vi "Run Explain Error.vi"(8 "error in (no error)":errorcluster, 11 "Data":errorcluster) -> (0 "error out":errorcluster)   [LabVIEW 2011, in "Simple Error Out.xctl"]
uses:
  Simple Error Out.xctl
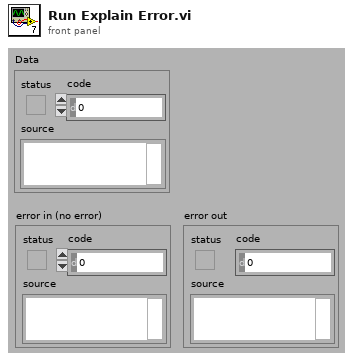
[diagram p1: front panel]
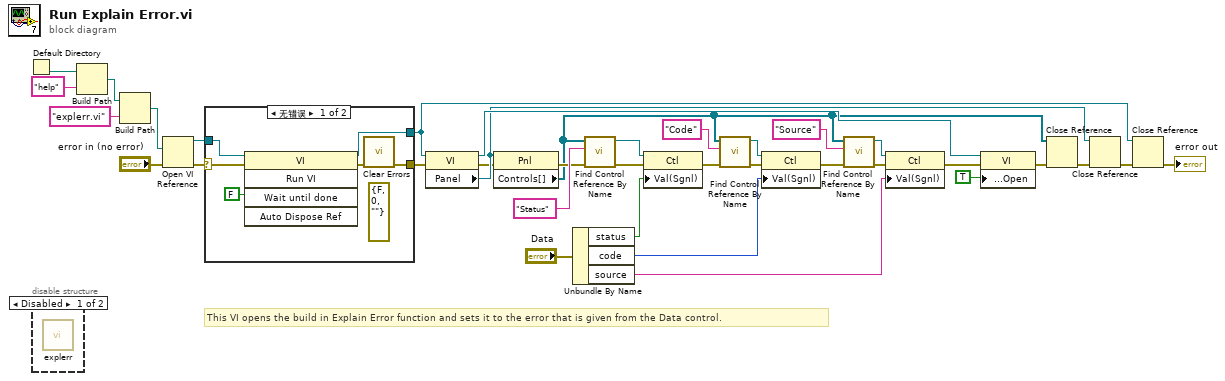
[diagram p0: block diagram]
diagram:
  # "This VI opens the build in Explain Error function and sets it to the error that is given from the Data control."
  n1 = Default Directory() -> (w36:path)
  n2 = disable-structure shown="Disabled" {
    frame Disabled {
      n3 = call <helpdir>:"explerr.vi"() -> ()  [unwired: 1 in, 1 out]
    }
    frame Enabled {
    }
  }
  n4 = Build Path(base path=w36, name or relative path="help") -> (appended path=w34:path)
  n5 = Build Path(base path=w34, name or relative path="explerr.vi") -> (appended path=w32:path)
  n6 = Open VI Reference(vi path=w32, error in (no error)="error in (no error)") -> (vi reference=w5:refnum<vi>, error out=w4:errorcluster)  [unwired: 4 in]
  n7 = case shown="无错误" w4 {
    selector: w4 -> [w40 w44]
    tunnel: w5 -> [w42 w43]
    tunnel: [w38 w44] -> w3
    tunnel: [w37 w43] -> w1
    frame No Error {
      (unwired) errorcluster {"status"=FALSE, "code"=0, "source"=""} ("error IO")
      n8 = invoke class="VI" method="Run VI"(reference=w42, error in=w40, "Wait until done"=FALSE ("Wait Until Done")) -> (reference out=w37:refnum<vi>, error out=w39:errorcluster)  [unwired: 2 in, 3 out]
      n9 = call <vilib>:"Clear Errors.vi"("error in (no error)"=w39) -> ("error out"=w38:errorcluster)  [unwired: 6 in]
    }
    frame Error {
    }
  }
  n10 = property class="VI"(reference=w1, error in=w3) -> (reference out=w31:refnum<vi>, error out=w6:errorcluster, "Panel"=w9:refnum<vi>)
  n11 = property class="Pnl"(reference=w9, error in=w6) -> (error out=w28:errorcluster, "Controls[]"=w10:refnum<vi>[])  [unwired: 1 out]
  n12 = Unbundle By Name("Data") -> ("status"=w24:bool, "code"=w19:i32, "source"=w14:string)
  n13 = call "Find Control Reference By Name.vi"("error in (no error)"=w28, "Name"="Status", "Controls[]"=w10) -> ("error out"=w26:errorcluster, "Ctl Refnum"=w27:refnum<vi>)  [unwired: 7 in]
  n14 = property class="Ctl"(reference=w27, error in=w26, "Val(Sgnl)"=w24) -> (error out=w20:errorcluster)  [unwired: 1 out]
  n15 = call "Find Control Reference By Name.vi"("error in (no error)"=w20, "Name"="Code", "Controls[]"=w10) -> ("error out"=w23:errorcluster, "Ctl Refnum"=w22:refnum<vi>)  [unwired: 7 in]
  n16 = property class="Ctl"(reference=w22, error in=w23, "Val(Sgnl)"=w19) -> (error out=w16:errorcluster)  [unwired: 1 out]
  n17 = call "Find Control Reference By Name.vi"("error in (no error)"=w16, "Name"="Source", "Controls[]"=w10) -> ("error out"=w17:errorcluster, "Ctl Refnum"=w18:refnum<vi>)  [unwired: 7 in]
  n18 = property class="Ctl"(reference=w18, error in=w17, "Val(Sgnl)"=w14) -> (error out=w13:errorcluster)  [unwired: 1 out]
  n19 = property class="VI"(reference=w31, error in=w13, "Front Panel.Open"=TRUE ("Front Panel Window:Open")) -> (error out=w2:errorcluster)  [unwired: 1 out]
  n20 = Close Reference(reference=w10, error in (no error)=w2) -> (error out=w12:errorcluster)
  n21 = Close Reference(reference=w9, error in (no error)=w12) -> (error out=w11:errorcluster)
  n22 = Close Reference(reference=w1, error in (no error)=w11) -> (error out=→"error out":errorcluster)
